vi "meteo_test.vi"() -> ()   [LabVIEW 2011]
panel:
  in  "QUIT":bool
  out "error out":errorcluster
  out "keyword":string
  out "data out":string
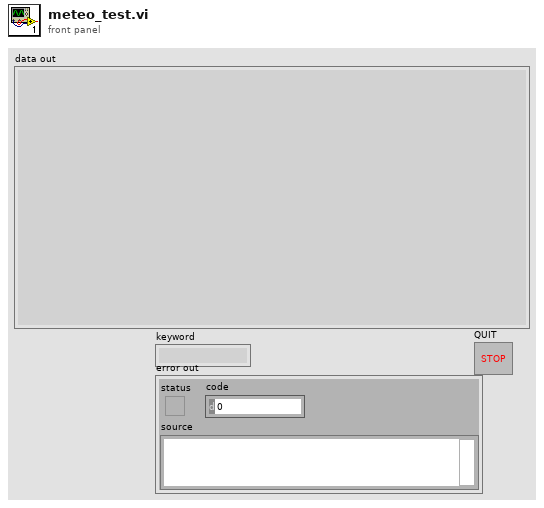
[diagram p1: front panel]
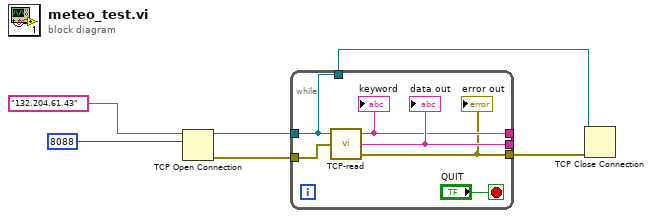
[diagram p0: block diagram]
diagram:
  n1 = TCP Open Connection(address="132.204.61.43", remote port or service name=u16 8088) -> (connection ID=w6:refnum<k5>, error out=w5:errorcluster)  [unwired: 3 in]
  n2 = while {
    tunnel: w6 -> [w7]
    tunnel: w5 -> [w12]
    tunnel: [w11] -> _
    tunnel: [w10] -> _
    tunnel: [w9] -> w2
    tunnel: [w7] -> w1
    stop <- "QUIT" stop-if-true
    n3 = call "TCP-read.vi"("error in (no error)"=w12, "connection ID"=w7) -> ("error out"=w9:errorcluster, "data out"=w11:string, "keyword"=w10:string)  [unwired: 1 in]
    "data out" <- w11
    "keyword" <- w10
    "error out" <- w9
  }
  n4 = TCP Close Connection(connection ID=w1, error in (no error)=w2) -> ()  [unwired: 1 in, 2 out]
